vi "AddNode.vi"(5 "VI":string, 9 "VI_AST in":refnum<class "VI_Hierarchy.lvclass">) -> (3 "VI_AST out":refnum<class "VI_Hierarchy.lvclass">, 4 "index":i32)   [LabVIEW 2014, in "VI_Hierarchy.lvclass"]
uses:
  VI_Hierarchy.lvclass
  VI_Hierarchy.lvclass/VI_Hierarchy.ctl
  DAG/DAG/DAG.lvclass
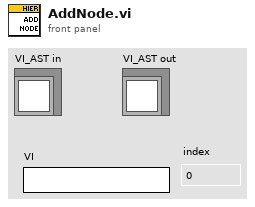
[diagram p1: front panel]
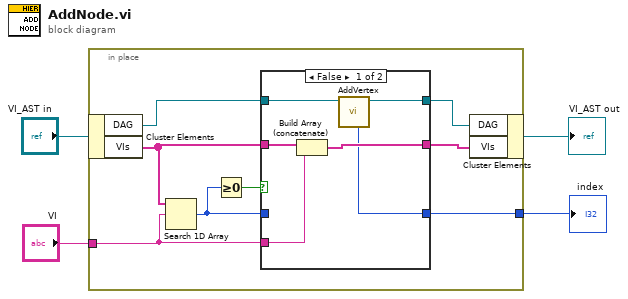
[diagram p0: block diagram]
diagram:
  n1 = in-place {
    in-place-border: "VI" -> [w9]
    in-place-border: [w8] -> w1
    n2 = in-place-cluster #1("VI_AST in") -> ("DAG"=w6:refnum<class "DAG.lvclass">, "VIs"=w11:string[])
    n3 = Search 1D Array(1D array=w11, element=w9) -> (index of element=w7:i32)  [unwired: 1 in]
    n4 = Greater Or Equal To 0?(x=w7) -> (x >= 0?=w12:bool)
    n5 = case shown="False" w12 {
      tunnel: w11 -> [w18 w21]
      tunnel: [w16 w21] -> w10
      tunnel: w9 -> [w17 _]
      tunnel: [w13 w20] -> w8
      tunnel: w7 -> [_ w20]
      tunnel: w6 -> [w15 w19]
      tunnel: [w14 w19] -> w5
      frame False {
        n6 = Build Array (concatenate)(w18, w17) -> (w16:string[])
        n7 = call "AddVertex.vi"("DAG in"=w15) -> ("DAG out"=w14:refnum<class "DAG.lvclass">, "vertex out"=w13:i32)  [unwired: 7 in]
      }
      frame True {
      }
    }
    n8 = in-place-cluster #1("DAG"=w5, "VIs"=w10) -> (→"VI_AST out":refnum<class "VI_Hierarchy.lvclass">)
  }
  "index" <- w1
